vi "update_tree.vi"(0 "当前项目UI.项目路径":path, 1 "项目管理UI":refnum<vi>, 3 "父项":string) -> ()   [LabVIEW 2018, in "menu.lvlib"]
uses:
  menu.lvlib
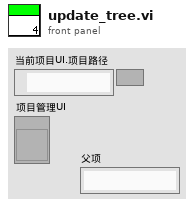
[diagram p1: front panel]
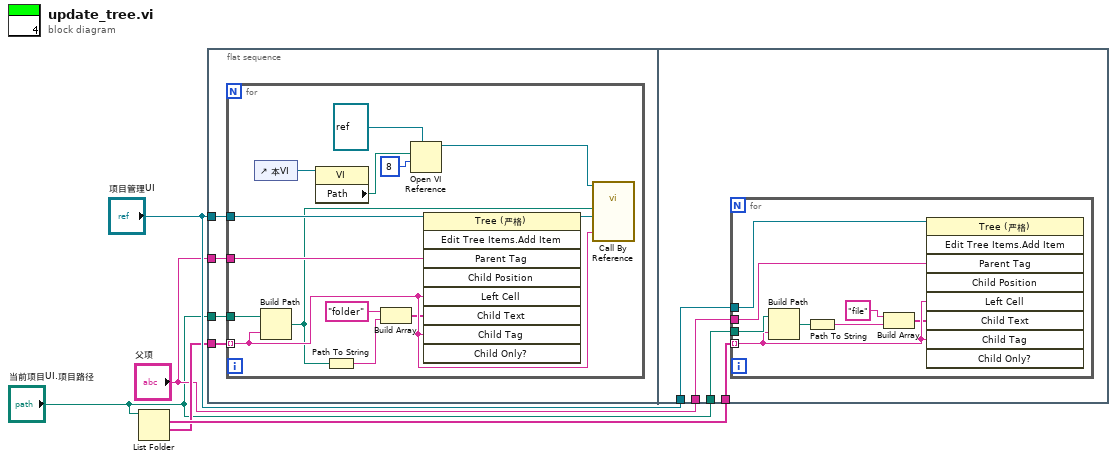
[diagram p0: block diagram]
diagram:
  n1 = List Folder(path="当前项目UI.项目路径") -> (filenames=w5:string[], folder names=w3:string[])  [unwired: 3 in, 2 out]
  n2 = flat-sequence {
    tunnel: w3 -> [w9]
    tunnel: "当前项目UI.项目路径" -> [w8]
    tunnel: "项目管理UI" -> [w7]
    tunnel: "父项" -> [w6]
    tunnel: w5 -> [w27]
    tunnel: "项目管理UI" -> [w26]
    tunnel: "父项" -> [w25]
    tunnel: "当前项目UI.项目路径" -> [w24]
    frame #0 {
      n3 = for {
        tunnel: w9 -> [w14] mode=indexing
        tunnel: w8 -> [w23]
        tunnel: w7 -> [w17]
        tunnel: w6 -> [w15]
        n4 = control-ref of="本VI"() -> (w22:refnum<vi>)
        n5 = Build Path(base path=w23, name or relative path=w14) -> (appended path=w12:path)
        n6 = property class="VI"(reference=w22) -> ("Path"=w21:path)  [unwired: 1 in, 2 out]
        n7 = Path To String(path=w12) -> (string=w13:string)
        n8 = Build Array("folder" ("元素"), w13) -> (w11:string[])
        n9 = Open VI Reference(type specifier VI Refnum (for type only)=refnum<vi> refnum ("类型说明符VI引用句柄（仅用于类型）"), vi path=w21, options=8 ("选项")) -> (vi reference=w20:refnum<vi>)  [unwired: 3 in, 1 out]
        n10 = invoke class="Tree (严格)" method="Edit Tree Items.Add Item"(reference=w17, "Parent Tag"=w15, "Left Cell"=w14, "Child Text"=w11, "Child Tag"=w14) -> (reference out=w16:refnum<vi>)  [unwired: 4 in, 8 out]
        n11 = call-by-ref "?"(reference=w20, "当前项目UI.项目路径"=w12, "项目管理UI"=w16, "父项"=w14) -> ()  [unwired: 9 in, 2 out]
      }
    }
    frame #1 {
      n12 = for {
        tunnel: w27 -> [w32] mode=indexing
        tunnel: w26 -> [w35]
        tunnel: w25 -> [w34]
        tunnel: w24 -> [w33]
        n13 = Build Path(base path=w33, name or relative path=w32) -> (appended path=w31:path)
        n14 = Path To String(path=w31) -> (string=w30:string)
        n15 = Build Array("file" ("元素"), w30) -> (w29:string[])
        n16 = invoke class="Tree (严格)" method="Edit Tree Items.Add Item"(reference=w35, "Parent Tag"=w34, "Left Cell"=w32, "Child Text"=w29, "Child Tag"=w32) -> ()  [unwired: 4 in, 9 out]
      }
    }
  }
